vi "Execute.vi"(8 "error in (no error)":errorcluster, 10 "System In":refnum<class "abs_System.lvclass">, 11 "Node in":refnum<class "Repeat Until Count.lvclass">) -> (0 "error out":errorcluster, 1 "Status":T1, 2 "System Out":refnum<class "abs_System.lvclass">, 3 "Node out":refnum<class "Repeat Until Count.lvclass">)   [LabVIEW 2021, in "BT.lvlib" / "Repeat Until Count.lvclass"]
uses:
  Repeat Until Count.lvclass
  abs_Node/Status.ctl
  abs_System/abs_System.lvclass
  Repeat Until Count.lvclass/Repeat Until Count.ctl
  Repeater/Repeater.lvclass
  abs_Node/abs_Node.lvclass
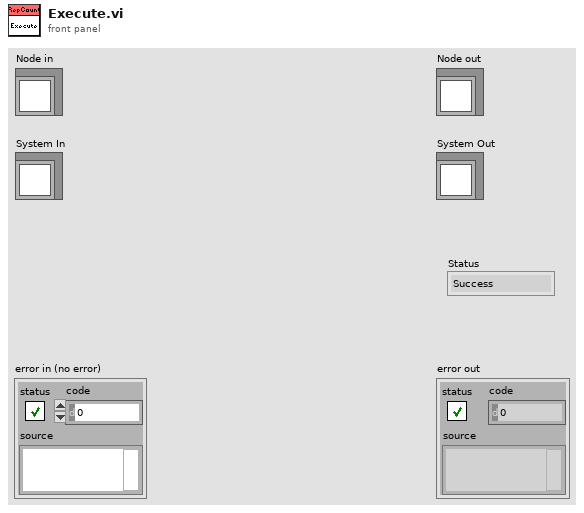
[diagram p1: front panel]
types:
  T1 = typedef "BT.lvlib/abs_Node.lvclass/Status.ctl" = enum16{"Success", "Failure", "Running"}
  T2 = typedef "BT.lvlib/Repeat Until Count.lvclass/On Count Status - Type.ctl" = enum16{"Success", "Failure"}
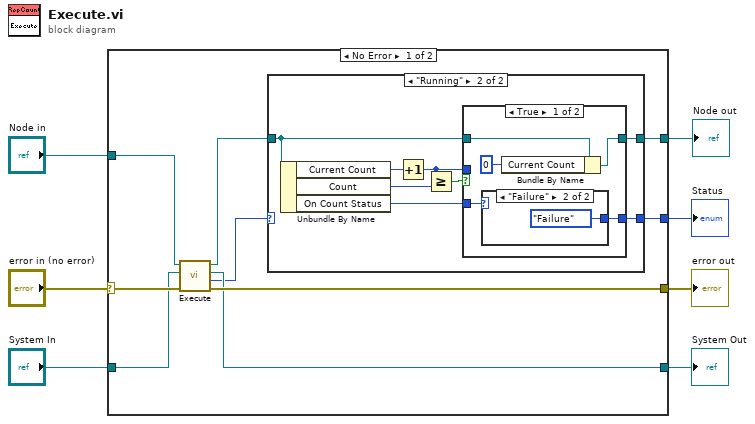
[diagram p0: block diagram]
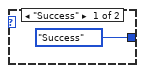
[diagram p3: hidden frame]
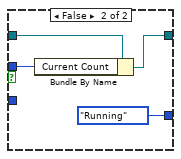
[diagram p4: hidden frame]
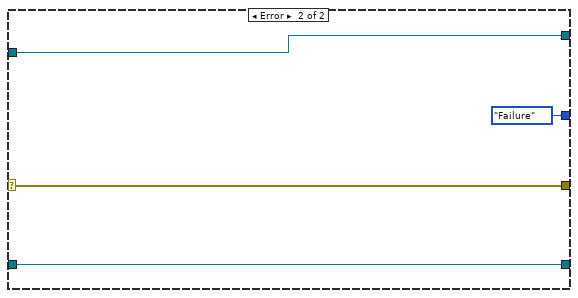
[diagram p5: hidden frame]
diagram:
  n1 = case shown="No Error" "error in (no error)" {
    selector: "error in (no error)" -> [w14 w39]
    tunnel: [w16 w39] -> w7
    tunnel: [w15 w38] -> w6
    tunnel: "System In" -> [w13 w38]
    tunnel: "Node in" -> [w12 w41]
    tunnel: [w9 Status."Failure" ("Status")] -> w2
    tunnel: [w8 w41] -> w1
    frame No Error {
      n2 = call-parent "Execute.vi"("error in (no error)"=w14, "System In"=w13, "Node in"=w12) -> ("error out"=w16:errorcluster, "Status"=w10:T1, "System Out"=w15:refnum<class "abs_System.lvclass">, "Node out"=w11:refnum<class "Repeat Until Count.lvclass">)  [unwired: 5 in]
      n3 = case shown="\"Running\"" w10 {
        selector: w10 -> [w18 _]
        tunnel: w11 -> [w17 w23]
        tunnel: [w18 w19] -> w9
        tunnel: [w17 w22] -> w8
        frame Default {
        }
        frame "Running" {
          n4 = Unbundle By Name(w23) -> ("Current Count"=w26:i32, "Count"=w25:i32, "On Count Status"=w20:T2)
          n5 = Increment(x=w26) -> (x+1=w21:i32)
          n6 = Greater Or Equal?(x=w21, y=w25) -> (x >= y?=w24:bool)
          n7 = case shown="True" w24 {
            tunnel: w23 -> [w31 w37]
            tunnel: [w30 w36] -> w22
            tunnel: w21 -> [_ w35]
            tunnel: w20 -> [w28 _]
            tunnel: [w27 Status."Running" ("Status")] -> w19
            frame True {
              n8 = case shown="\"Failure\"" w28 {
                tunnel: [Status."Success" ("Status") Status."Failure" ("Status")] -> w27
                frame "Success" {
                }
                frame "Failure" {
                }
              }
              n9 = Bundle By Name(cluster=w31, "Current Count"=0) -> (w30:refnum<class "Repeat Until Count.lvclass">)
            }
            frame False {
              n10 = Bundle By Name(cluster=w37, "Current Count"=w35) -> (w36:refnum<class "Repeat Until Count.lvclass">)
            }
          }
        }
      }
    }
    frame Error {
    }
  }
  "error out" <- w7
  "Node out" <- w1
  "Status" <- w2
  "System Out" <- w6
